vi "ProdaNG.Example.GetTestSteps.vi"() -> ()   [LabVIEW 2016]
uses:
  Controls/ProdaNG.Identification.ctl
  Controls/ProdaNG.TestStep.ctl
  Controls/ProdaNG.ProcessStep.ctl
  Controls/ProdaNG.Process.ctl
  Controls/ProdaNG.ProcessStepParam.ctl
  <vilib>/Utility/miscctls.llb/LVRowAndColumnUnsignedTypeDef.ctl
panel:
  in  "ResultStatus":i32(listbox)
  out "Identification":T1
  in  "ButtonUpdate":bool
  in  "ButtonRead":bool
  in  "Results":i32(listbox)
  out "ProcStepParams":T2[](array[typedef])
  out "Process":T3
  out "ProcStep":T4[](array[typedef])
  out "TestSteps":T5[](array[typedef])
  in  "Product Serial Number":string="1160131100027"
  out "ID":T6
  in  "Systems":u16(ring) items=["ADEK1", "ASTV2_P01", "ASTV2_P02", "ASTV2_P03", "ASTV2_P04", "Connection station", "DPI", "EAPU2_AD", "EAPU2_CONN", "EAPU2_MCPV_1", "EAPU2_MCPV_2", "EBAM2", "EBAM3", "EBAM4", "ED01", "ED04", "ED05", "EPS3_RANGE_DMC", "FAVP_1A", "FAVP_1B", "FESTO", "H17", "H20", "H21", "HAPU P01", "HAPU P02", "HAPU P03", "HAPU_P01", "HAPU_P02", "HAPU_P03", "HAPU_P04", "HAPU_P05", "HAPU_P06", "HP1", "HP10", "HP10L", "HP10R", "HP12", "HP13", "HP15", "HP16", "HP17", "HP18", "HP19", "HP2", "HP20", "HP21", "HP22", "HP23", "HP24", "HP25", "HP26", "HP26L", "HP26R", "HP2L", "HP2R", "HP3", "HP34", "HP35", "HP37", "HP38", "HP39", "HP4", "HP50", "HP51", "HP52", "HP6", "HP7", "HP8", "HP88", "HP8L", "HP8R", "HP9", "KEPSE1", "KEPSE2", "KEPSE3", "KEPSE4", "KEPSE5", "LCS02", "LSM101", "LSM102", "LSM103", "LV_MIX_process", "MAD 1.A", "MAD 1.B", "MAD 2.B", "MAD 2.C", "MAD 4.A", "MAD 4.B", "MAD EOL", "MIX_400", "MIX_820", "MIX_821", "MIX_BST3_030", "MIX_BST3_034", "MT001", "MT002", "MT003", "MT004", "MT005", "MT006", "MT009", "MT010", "MT011", "MT012", "MT013", "MT014", "MT015", "MT016", "MT017", "MT018", "MT019", "MT020", "MT021", "MT022", "MT023", "MT024", "MT025", "MTB1", "MTB10", "MTB11", "MTB12", "MTB14", "MTB15", "NI_06", "NI_13", "P01", "P02", "P25", "P25L", "P25R", "P32", "P32L", "P34", "PEPS3Gang1", "PEPS3Gang2", "PLATES1", "PLC01", "PLC01L", "PLC01R", "PLC02", "PLC02L", "PLC02R", "PLC03", "PLC04", "PLC04L", "PLC04R", "PLC06L", "PLC06R", "PLC07", "PLC07L", "PLC07R", "PLC08", "PLC08L", "PLC08R", "PLC09", "PLC09L", "PLC09R", "PLC10", "PLC11", "PLC11L", "PLC11R", "PLC12", "PLC12L", "PLC12R", "PLC13", "PLC13L", "PLC13R", "PLC14", "PLC14L", "PLC14R", "PLC15", "PLC15L", "PLC15R", "PLC16", "PLC16L", "PLC16R", "PLC17", "PLC17L", "PLC17R", "PLC18", "PLC19", "PLC19L", "PLC19R", "PLC20", "PLC21", "PLC22", "PLC23", "PLC24", "PLC25", "PLC254", "PLC25L", "PLC25R", "PLC27", "PLC27L", "PLC27R", "PLC28", "PLC28L", "PLC28R", "PLC29", "PLC29L", "PLC29R", "PLC30", "PLC31", "PLC32", "PLC34L", "PLC34R", "PLC36", "PLC38", "PLC39", "PLC39L", "PLC39R", "PLC40", "PLC40L", "PLC40R", "PLC41", "PLC41L", "PLC41R", "PLC42", "PLC42L", "PLC42R", "PLC43", "PLC44", "PLC44L", "PLC44R", "PLC45", "PLC45L", "PLC45R", "PLC46", "PLC46L", "PLC46R", "PSPS_02", "RAVP_1", "RAVP_100", "RAVP_2", "RAVP_3", "RIG1", "RIG10", "RIG110", "RIG111", "RIG13", "RIG14", "RIG150", "RIG151", "RIG160", "RIG161", "RIG17", "RIG18", "RIG19", "RIG2", "RIG20", "RIG21", "RIG22", "RIG23", "RIG24", "RIG26", "RIG27", "RIG271", "RIG272", "RIG28", "RIG29", "RIG291", "RIG292", "RIG3", "RIG30", "RIG31", "RIG32", "RIG321", "RIG322", "RIG33", "RIG331", "RIG332", "RIG34", "RIG4", "RIG5", "RIG6", "RIG7", "RIG80", "RIG90", "RSS_PLUS_BASIC_05", "RSS_PLUS_BASIC_P01", "RSS_PLUS_BASIC_S02", "SD001", "SD002", "SMV1_A", "SMV1_B", "SMV2_A", "SMV2_B", "SMV_017300_1", "SMV_017300_2", "SMV_021300_1", "SMV_021300_2", "SMV_320_1", "SMV_320_2", "T001", "T002", "T003", "T004", "T005", "T006", "T007", "T008", "T009", "T010", "T011", "T012", "T013", "T014", "T015", "T016", "T017", "T018", "T019", "T020", "T021", "T022", "T023", "T023_1", "T024", "T025", "T026", "T027", "T028", "T029", "T030", "T031", "T032", "T033", "T034", "T035", "T036", "T037", "T038", "T039", "T040", "T041", "T042", "T043", "T044", "T045", "T050", "T051", "T052", "T053", "T054", "T055", "T056", "T057", "T058", "T059", "T060", "T061", "T062", "T063", "T064", "T065", "T066", "T067", "T068", "T069", "T070", "T071", "T072", "T073", "T074", "T075", "T076", "T077", "T078", "T079", "T080", "T081", "T082", "T083", "T084", "T085", "T086", "T087", "T088", "T089", "T090", "T091", "T092", "T093", "T094", "T095", "T096", "T209", "TB01", "TB02", "TB_MTB59", "TB_MTB60", "TCSVCS_P01", "TCSVCS_P02", "TCSVCS_P03", "TCSVCS_P04", "TEBS-E_01", "TEBS-E_02", "TEBS-E_03", "TEBS-E_04", "TEBS-E_05", "TEBS-E_06A", "TEBS-E_06B", "TEBS-E_06C", "TEBS-E_07", "TEBS-E_08", "TEBS-E_09", "TEBS-E_F_P01", "TEBS-E_F_P02", "TEBS-E_F_P03", "TEBS-E_L_P01", "TEBS-E_L_P02", "TEBS-E_L_P03", "TEBS-P01", "TEBS-P02", "TEBS-P03", "TEBS_OT_P1", "TEBS_OT_P2", "TO29", "T_REMAN_COMP_1", "VXI15", "YR1_T001", "YR1_T002", "YR1_T003", "YR1_T004", "YR1_T005", "YR1_T006", "YR1_T007", "YR1_T008", "YR1_T009", "YR1_T010", "YR1_T011", "YR1_T012", "YR1_T013", "YR1_T014", "YR1_T015", "YR1_T016", "unknown"]
  in  "Wabco Number":u16(ring)=3155 items=["0", "0000000002", "0000000003", "0000000004", "0000000005", "0000000009", "0000000010", "0000000012", "0000000013", "0000000091", "0000000092", "0000000093", "0000000094", "0000000095", "0000000111", "0000000112", "0000000113", "0000000910", "0000000911", "0000000920", "0000000921", "0000000923", "0000000930", "0000000931", "0000000940", "0000000990", "0000000991", "0000000992", "1001001009", "1100000000", "1111110610", "1111111110", "1111111111", "1111111112", "1111111113", "1111111114", "1111111115", "1111111116", "1111111117", "1111111119", "1111111150", "1111111190", "1111118050", "1111119999", "1201201200", "1231231230", "1231231231", "1231231232", "1234567890", "1324070012", "1324079202", "1347141250", "2111111111", "2211111111", "2220009980", "2220009990", "2220110090", "2221111111", "2222222220", "2222222221", "2222222222", "2222222230", "2222222250", "2222222260", "2222222310", "2222222320", "2222222360", "2222222410", "2222222430", "2222222490", "2222223330", "2222224440", "2222225000", "2222510030", "2222510070", "2222510080", "2222510090", "2347141250", "3111111110", "3240020010", "3240020160", "3240020210", "3240026660", "3330110000", "3330110010", "3333333331", "3333333333", "3401750002", "3401950002", "3402250002", "3720600220", "3720600620", "3730110000", "3730110010", "3730110020", "3730110030", "3730110040", "3730110050", "3730110060", "3730110070", "3730110080", "3730110090", "3750103000", "3750103010", "3750103020", "3750103140", "3750103170", "3750103180", "3750103320", "3750103330", "3750150040", "3750150050", "3750150260", "3750150680", "3750150720", "3750150730", "3750155120", "4005000700", "4005000707", "4005000810", "4005000817", "4005000820", "4005000828", "4005000830", "4005000870", "4005000880", "4005001020", "4005001030", "4005001050", "4005001111", "4005009252", "4005009999", "4006000100", "4111510090", "4111510092", "4111540040", "4111540042", "4123520162", "4123520270", "4123520272", "4123520300", "4123520302", "4127040010", "4127040040", "4127040050", "4127040080", "4127040087", "4127040089", "4127040090", "4127040130", "4127040132", "412704013R", "4127040150", "4127040159", "4127040180", "4127040230", "4127040240", "4127040242", "4127040270", "4127040272", "4129990114", "4129990115", "4129990118", "4129990125", "4129990135", "4129990145", "4129990175", "4129990185", "4129990305", "4129990325", "4129990335", "4129990504", "4129996252", "4129996504", "4129996604", "4129996614", "4129996804", "4129996814", "4129996824", "4129996834", "4129996844", "4129996854", "4129996904", "4129996914", "4129996924", "4129997302", "4129997312", "4129997322", "4129998002", "4129999504", "4129999524", "4154043122", "4213500010", "4213500610", "4213500720", "4213500800", "4213500810", "4213500820", "4213500830", "4213500840", "4213500850", "4213500860", "4213500870", "4213500880", "4213509272", "4213509282", "4213509302", "4213509312", "4213509322", "4213509342", "4213509352", "4213509930", "4213509999", "4213510000", "4213510010", "4213510510", "4213510700", "4213510750", "4213510960", "4213510970", "4213510980", "4213511300", "4213511310", "4213511320", "4213511330", "4213511350", "4213511360", "4213511370", "4213511380", "4213511400", "4213511440", "4213511510", "4213511520", "4213511530", "4213511540", "4213511550", "4213511560", "4213511650", "4213511660", "4213511670", "4213511710", "4213511719", "4213511720", "4213511730", "4213511740", "4213511750", "4213511760", "4213511770", "4213511780", "4213511790", "4213511840", "4213511860", "4213511870", "4213519382", "4213519392", "4213519402", "4213519980", "4213519990", "4213520820", "4213529202", "4213529800", "4213529880", "4213529900", "4213529910", "4213529920", "4213529930", "4213529940", "4213529950", "4213529960", "4213529970", "4213529980", "4213529990", "4213554524", "4213554532", "4214113000", "4214113010", "4214113020", "4214113040", "4214113050", "4214113060", "4214113080", "4214113090", "4214113110", "4214113140", "4214113150", "4214113160", "4214150022", "4214270002", "4214290020", "4214290030", "4214290050", "4214290060", "4214410002", "4214410030", "4214410130", "4214410200", "4214410500", "4214410600", "4214420000", "4214420002", "4214420080", "4214420130", "4214420170", "4214420180", "4214420530", "4228020134", "4228023010", "4228023018", "4228023090", "4228023098", "4228023100", "4228023108", "4228023200", "4228023208", "4228023250", "4228023258", "4228023260", "4228024020", "4228024210", "4228024218", "4228033270", "4228033280", "4228033288", "4228081060", "4228081068", "4228090002", "4228100002", "4228100012", "4228100022", "4228100032", "4228110002", "4228120000", "4228120002", "4228120008", "4228120020", "4228120028", "4228120104", "4228120114", "4229010164", "4229020104", "4229030134", "4229030164", "4230000000", "4230035020", "4230035080", "4230039110", "4230070190", "4230080050", "4230080070", "4230089160", "4230089170", "4230089190", "4230540000", "4230540010", "4230550000", "4230550010", "4230550060", "4230550080", "4230550500", "4230550530", "4230551000", "4230560000", "4230560010", "4230560040", "4230560060", "4230560080", "4230560500", "4230560530", "4230570002", "4230570010", "4230570030", "4230570070", "4230570080", "4230570100", "4230580010", "4230580020", "4230600000", "4230600040", "4231020120", "4231020150", "4231029000", "4231030050", "4231030100", "4231031000", "4231031180", "4231032960", "4231032980", "4231039000", "4231040020", "4231040060", "4231040070", "4231040100", "4231040200", "4231040500", "4231040530", "4231040930", "4231040990", "4231042910", "4231042980", "4231046060", "4231046070", "4231046080", "4231046100", "4231046120", "4231046130", "4231046180", "4231046300", "4231046310", "4231046320", "4231046340", "4231046350", "4231046360", "4231046530", "4231047000", "4231047010", "4231047100", "4231047110", "4231047120", "4231047130", "4231047150", "4231047160", "4231050040", "4231050200", "4231050210", "4231050220", "4231050310", "4231050320", "4231050420", "4231050430", "4231050720", "4231050740", "4231050840", "4231050850", "4231050890", "4231050910", "4231050940", "4231051030", "4231051110", "4231051180", "4231051210", "4231051230", "4231051250", "4231051260", "4231051300", "4231051310", "4231051340", "4231051350", "4231051990", "4231052920", "4231052960", "4231052970", "4231052980", "4231054060", "4231054070", "4231054080", "4231054090", "4231054100", "4231054140", "4231054160", "4231054170", "4231054500", "4231054510", "4231057000", "4231057010", "4231057020", "4231057030", "4231057040", "4231057050", "4231060020", "4231060030", "4231060040", "4231060050", "4231060410", "4231060460", "4231060470", "4231060570", "4231060580", "4231060700", "4231060710", "4231060810", "4231060880", "4231060900", "4231060950", "4231061030", "4231061040", "4231061060", "4231061150", "4231061180", "4231061250", "4231061260", "4231061300", "4231061350", "4231061360", "4231061440", "4231061500", "4231061510", "4231061520", "4231061600", "4231061700", "4231062010", "4231062020", "4231062070", "4231062080", "4231062100", "4231062920", "4231062930", "4231062940", "4231062950", "4231062970", "4231062980", "4231064020", "4231064030", "4231064060", "4231064070", "4231064080", "4231064090", "4231064100", "4231064170", "4231064210", "4231064220", "4231064230", "4231064260", "4231064280", "4231064300", "4231064500", "4231067000", "4231067010", "4231069050", "4231069250", "4231069260", "4231069320", "4231069600", "4231070070", "4231070080", "4231070100", "4231070310", "4231070320", "4231070500", "4231070600", "4231070900", "4231070980", "4231071110", "4231071120", "4231072980", "4231074020", "4231074030", "4231074040", "4231074060", "4231074070", "4231074080", "4231074100", "4231074110", "4231074160", "4231074170", "4231079220", "4231079300", "4231090010", "4231090020", "4231090030", "4231090070", "4231090080", "4231090100", "4231090130", "4231090200", "4231090220", "4231090230", "4231090700", "4231091010", "4231091020", "4231091180", "4231091200", "4231097000", "4231097010", "4231099000", "4231100010", "4231107100", "4231107110", "4231127100", "4231140000", "4231140010", "4231140020", "4231140030", "4231140080", "4231140100", "4231140110", "4231140300", "4231140400", "4231146000", "4231146100", "4231147100", "4232051000", "4232051010", "4232051050", "4232051060", "4232067000", "4232067010", "4235030000", "4235030010", "4235030100", "4235030110", "4235031800", "4235031810", "4235040010", "4235040020", "4235040030", "4235040120", "4235040130", "4235040140", "4235040200", "4235040210", "4235040240", "4235040300", "4235040810", "4235040900", "4235040910", "4235041000", "4235041010", "4235041100", "4235041300", "4235041800", "4235041810", "4235050000", "4235050010", "4235050020", "4235050040", "4235050070", "4235050080", "4235050140", "4235050150", "4235050200", "4235050210", "4235050220", "4235050230", "4235050240", "4235050500", "4235050510", "4235050600", "4235050610", "4235051800", "4235051810", "4235051900", "4235051910", "4235060010", "4235060020", "4235060030", "4235060060", "4235060070", "4235060080", "4235060090", "4235060140", "4235060150", "4235060200", "4235060210", "4235060220", "4235060230", "4235060240", "4235060250", "4235060260", "4235060270", "4235060310", "4235060400", "4235060420", "4235060430", "4235060500", "4235060501", "4235060510", "4235060520", "4235060530", "4235060540", "4235060550", "4235060560", "4235060570", "4235060600", "4235060610", "4235060620", "4235060630", "4235060640", "4235060650", "4235060720", "4235060810", "4235061000", "4235061010", "4235061020", "4235061030", "4235061040", "4235061041", "4235061200", "4235061210", "4235061220", "4235061230", "4235061240", "4235061300", "4235061310", "4235061400", "4235061401", "4235061410", "4235061420", "4235061430", "4235061431", "4235061500", "4235061510", "4235061600", "4235061610", "4235070000", "4235090050", "4235090060", "4235090070", "4235090080", "4235090100", "4235090110", "4235090120", "4235090130", "4235090200", "4235090210", "4235090220", "4235090230", "4235090240", "4235090250", "4235090260", "4235100010", "4235100100", "4235100200", "4235100210", "4235100240", "4235100250", "4235100260", "4235110100", "4235110110", "4235120010", "4235120100", "4235121800", "4235121810", "4235140000", "4235140030", "4235140040", "4235140060", "4235140100", "4235140200", "4321111111", "4324060012", "4324060022", "4324060032", "4324062222", "4324069202", "4324100000", "4324100002", "4324100012", "4324100022", "4324100030", "4324100040", "4324100042", "4324100050", "4324100052", "4324100070", "4324100080", "4324100200", "4324100210", "4324100220", "4324100230", "4324100260", "4324100270", "4324100310", "4324100330", "4324100340", "4324100350", "4324100360", "4324100380", "4324100410", "4324100420", "4324100500", "4324100640", "4324100660", "4324100670", "4324100690", "4324100720", "4324100730", "4324100740", "4324100750", "4324100760", "4324100790", "4324100800", "4324100830", "4324100870", "4324100900", "4324100910", "4324100920", "4324100950", "4324101020", "4324101040", "4324101060", "4324101100", "4324101110", "4324101120", "4324101130", "4324101140", "4324101150", "4324101160", "4324101170", "4324101180", "4324101200", "4324101210", "4324101220", "4324101230", "4324101270", "4324101310", "4324101340", "4324101350", "4324101440", "4324101620", "4324101660", "4324101670", "4324101910", "4324101920", "4324102000", "4324102010", "4324102020", "4324102040", "4324102160", "4324102210", "4324102500", "4324102620", "4324105522", "4324107200", "4324107350", "4324109070", "4324109312", "4324109322", "4324109332", "4324109352", "4324111600", "4324111670", "4324111680", "4324111690", "4324120010", "4324120020", "4324120030", "4324120040", "4324130010", "4324130020", "4324130030", "4324130060", "4324130070", "4324130090", "4324130300", "4324130320", "4324130330", "4324130660", "4324131020", "4324139202", "4324139232", "4324139242", "4324139252", "4324139292", "4324139302", "4324139312", "4324139322", "4324139332", "4324139342", "4324139999", "4324150000", "4324150002", "4324150030", "4324150050", "4324150060", "4324150080", "4324150090", "4324150100", "4324150120", "4324150130", "4324150150", "4324150160", "4324150170", "4324150190", "4324150220", "4324150240", "4324150280", "4324150290", "4324150300", "4324150320", "4324150330", "4324150370", "4324150380", "4324150390", "4324150500", "4324150590", "4324150620", "4324150690", "4324150720", "4324151240", "4324151380", "4324159210", "4324160010", "4324160020", "4324160030", "4324160040", "4324160110", "4324161110", "4324162220", "4324200000", "4324200020", "4324200030", "4324200080", "4324209202", "4324209212", "4324209222", "4324209242", "4324209252", "4324209262", "4324210000", "4324210002", "4324210020", "4324210030", "4324210070", "4324210080", "4324210090", "4324210100", "4324210110", "4324210120", "4324210140", "4324210190", "4324210200", "4324210210", "4324210220", "4324210240", "4324210250", "4324210260", "4324210280", "4324210290", "4324210300", "4324210320", "4324210340", "4324210350", "4324210370", "4324210380", "4324210390", "4324211280", "4324216666", "4324219202", "4324250070", "4324250080", "4324250090", "4324250100", "4324252000", "4324259202", "4324259212", "4324259222", "4324259232", "4324259242", "4324260010", "4324260110", "4324261110", "4324262220", "4324300022", "4324309202", "4324309232", "4324309242", "4324309252", "4324309262", "4324309272", "4324309492", "4324310002", "4324310022", "4324315512", "4324319232", "4324319242", "4324319252", "4324319302", "4324319312", "4324319322", "4324319332", "4324319342", "4324319352", "4324319362", "4324319372", "4324319382", "4324319402", "4324319422", "4324320002", "4324320012", "4324330020", "4324330030", "4324330050", "4324330060", "4324330070", "4324330080", "4324330090", "4324330100", "4324330110", "4324330120", "4324330130", "4324330140", "4324330180", "4324330200", "4324330220", "4324330230", "4324330240", "4324330620", "4324331080", "4324331110", "4324331120", "4324331130", "4324331910", "4324332000", "4324332010", "4324332016", "4324332020", "4324332050", "4324332060", "4324332090", "4324332170", "4324332180", "4324332190", "4324332200", "4324332230", "4324332250", "4324332730", "4324332740", "4324332780", "4324332790", "4324332800", "4324332810", "4324332960", "4324332970", "4324332980", "4324332990", "4324332997", "4324336667", "4324337770", "4324339202", "4324339212", "4324339222", "4324339232", "4324339242", "4324339990", "4324339997", "4341000000", "4341000200", "4341000209", "4341000210", "4341000220", "4341000230", "4341000240", "4341000250", "4341000260", "4341000270", "4341000280", "4341000290", "4341000320", "4341000330", "4341000339", "4341000340", "4341000349", "4341000350", "4341000370", "4341000380", "4341000390", "4341000430", "4341000470", "4341000479", "4341000480", "4341000489", "4341000490", "4341000499", "4341000510", "4341000519", "4341000800", "4341000820", "4341000830", "4341001170", "4341001210", "4341001219", "4341001220", "4341001229", "4341001230", "4341001239", "4341001240", "4341001249", "4341001250", "4341001259", "4341001260", "4341001269", "4341001270", "4341001279", "4341001280", "4341001289", "4341001300", "4341001301", "4341001305", "4341001309", "4341001310", "4341001319", "4341001330", "4341001360", "4341001390", "4341001430", "4341001440", "4341001449", "4341001500", "4341001510", "4341001520", "4341001530", "4341002110", "4341002200", "4341002210", "4341002220", "4341002230", "4341002240", "4341002250", "4341002260", "4341002270", "4341002279", "4341002280", "4341002289", "4341002290", "4341002300", "4341002309", "4341002310", "4341002320", "4341002329", "4341002330", "4341002340", "4341002349", "4341002350", "4341002360", "4341002430", "4341002440", "4341002450", "4341002460", "4341002490", "4341002499", "4341002510", "4341002530", "4341002539", "4341002540", "4341002560", "4341002570", "4341002590", "4341002600", "4341002610", "4341002620", "4341005040", "4341005050", "4341005070", "4341005080", "4341006000", "4341006010", "4341006020", "4341006030", "4341006039", "4341006040", "4341008880", "4341009900", "4341009910", "4341009970", "4341009990", "4341080000", "4342050012", "4342050210", "4342050260", "4342050270", "4342050280", "4342050300", "4342050310", "4342050320", "4342050330", "4342050500", "4342050510", "4342050600", "4342050610", "4342059980", "4342059990", "4429987202", "4444444444", "4445010000", "4445010010", "4445010040", "4460806062", "4460806072", "4461080850", "4461082010", "4461082040", "4461082060", "4461082080", "4461451154", "4461451222", "4461451223", "4461640220", "4461640340", "4462600202", "4469990002", "4469990012", "4469990042", "4469990052", "4528020000", "4600000001", "4600000002", "4600000003", "4610000000", "4610000010", "4610000030", "4610000110", "4610000120", "4610000160", "4610001110", "4611060002", "4611061000", "4611061020", "4611061027", "4611061060", "4611064780", "4611110000", "4611110002", "4611110010", "4611110020", "4611130010", "4613070022", "4613070042", "4613072000", "4613072007", "4613072020", "4613073990", "4613074190", "4613074390", "4613074580", "4613074670", "4613074750", "4613074757", "4613074790", "4613074797", "4613075200", "4613075210", "4613103620", "4613105500", "4613150000", "4613150010", "4613150020", "4613150022", "4613150030", "4613150032", "4613150033", "4613150040", "4613150041", "4613150042", "4613150052", "4613150060", "4613150070", "4613150080", "4613150120", "4613150140", "4613150170", "4613150180", "4613150190", "4613150210", "4613150220", "4613150260", "4613150270", "4613150340", "4613150360", "4613150410", "4613150420", "4613150430", "4613150440", "4613150470", "4613150480", "4613150490", "4613150500", "4613150520", "4613150530", "4613150550", "4613150580", "4613150590", "4613150600", "4613150610", "4613150630", "4613150640", "4613150650", "4613150680", "4613150690", "4613150700", "4613150710", "4613150730", "4613150740", "4613150760", "4613150770", "4613150780", "4613150820", "4613150830", "4613150860", "4613150890", "4613151070", "4613151500", "4613151510", "4613151530", "4613151540", "4613151550", "4613151610", "4613151800", "4613152390", "4613152450", "4613152500", "4613152530", "4613152540", "4613152580", "4613152610", "4613152630", "4613152640", "4613154430", "4613154500", "4613154550", "4613154590", "4613154600", "4613154610", "4613154630", "4613154640", "4613154670", "4613154700", "4613154760", "4613154790", "4613154820", "4613154860", "4613154890", "4613154900", "4613154910", "4613154950", "4613154951", "4613154970", "4613155000", "4613159022", "4613159042", "4613159052", "4613159062", "4613159072", "4613159082", "4613159092", "4613159142", "4613159152", "4613159162", "4613159172", "4613159182", "4613159202", "4613159212", "4613159222", "4613159232", "4613159242", "4613159252", "4613159262", "4613159272", "4613159302", "4613159312", "4613159322", "4613159332", "4613160020", "4613180000", "4613180010", "4613180020", "4613180030", "4613180050", "4613180060", "4613180090", "4613180140", "4613180150", "4613180160", "4613180190", "4613180220", "4613180230", "4613180240", "4613180250", "4613180260", "4613180280", "4613180290", "4613180300", "4613180340", "4613180350", "4613180360", "4613180380", "4613180400", "4613180470", "4613180490", "4613180500", "4613180510", "4613180530", "4613180560", "4613180570", "4613180580", "4613180590", "4613180700", "4613180710", "4613181010", "4613184850", "4613184860", "4613184940", "4613184950", "4613185010", "4613185020", "4613185030", "4613185500", "4613185510", "4613185520", "4613186010", "4613186030", "4613186038", "4613186040", "4613186048", "4613186050", "4613186060", "4613186090", "4613186098", "4613186110", "4613189202", "4613189212", "4613189222", "4613189242", "4613189252", "4613190012", "4613190022", "4613190032", "4613190042", "4613190052", "4613190062", "4613190072", "4613190080", "4613190082", "4613190092", "4613190110", "4613190180", "4613190280", "4613190320", "4613190880", "4613192500", "4613192600", "4613192620", "4613192630", "4613192640", "4613192700", "4613192710", "4613192720", "4613192730", "4613192740", "4613192750", "4613192800", "4613199002", "4613199012", "4613199022", "4613199032", "4613199052", "4613199072", "4613199082", "4613199092", "4613199102", "4613199112", "4613199122", "4613240002", "4613240010", "4613240060", "4613240080", "4613240090", "4613240120", "4613240180", "4613240187", "4613240220", "4613240270", "4613240310", "4613240340", "4613240390", "4613240400", "4613240410", "4613240420", "4613240430", "4613240460", "4613245200", "4613245220", "4613246202", "4613280000", "4613300030", "4613330000", "4614780000", "4614780070", "4614820110", "4614820120", "4614820130", "4614820950", "4614911007", "4614911020", "4614911027", "4614911580", "4614911587", "4614912740", "4614912747", "4614940130", "4614947000", "4614947010", "4614947020", "4614947030", "4614947040", "4614947050", "4614947060", "4614947070", "4614947080", "4614990002", "4614990050", "4615130000", "4615130007", "4615130008", "4615130009", "4615130010", "4615130019", "4615130020", "4615130027", "4615130028", "4615130030", "4615130090", "4615130100", "4615130200", "4615130210", "4615130211", "4615130212", "4615130219", "4615131111", "4615139000", "4615139010", "4615139212", "4615139222", "4615139998", "4615139999", "4621930012", "4630220200", "4630220210", "4630281120", "4630281130", "4630320012", "4630320200", "4630320220", "4630320230", "4630320260", "4630320290", "4630321200", "4630321260", "4630321300", "4630321360", "4630380002", "4630380030", "4630380090", "4630380110", "4630380120", "4630380130", "4630380150", "4630390002", "4630390050", "4630390060", "4630489202", "4630489212", "4630840000", "4630840002", "4630840007", "4630840012", "4630840020", "4630840022", "4630840030", "4630840100", "4630840105", "4630840107", "4630840109", "4630840200", "4630840207", "4630840208", "4630840209", "4630840290", "4630840310", "4630840311", "4630840317", "4630840318", "4630840319", "4630840410", "4630840419", "4630840420", "4630840429", "4630840500", "4630840509", "4630841000", "4630841005", "4630841009", "4630849202", "4630849999", "4630860000", "4630860010", "4630860200", "4630860210", "4630860220", "4630860230", "4630860240", "4630860400", "4630860410", "4630860430", "4630860600", "4630860610", "4630900100", "4630900120", "4630900200", "4630900201", "4630900208", "4630900209", "4630900210", "4630900220", "4630900230", "4630900232", "4630900237", "4630900238", "4630900239", "4630900250", "4630901230", "4630905000", "4630905010", "4630905020", "4630905030", "4630905040", "4630905050", "4630905090", "4630905091", "4630905092", "4630905098", "4630905100", "4630999999", "4640060000", "4640060002", "4640060007", "4640060010", "4640060012", "4640060020", "4640060027", "4640060030", "4640060040", "4640060050", "4640060060", "4640060070", "4640060110", "4640060120", "4640060127", "4640060128", "4640060130", "4640061000", "4640061007", "4640061010", "4640061018", "4640061020", "4640062010", "4640065000", "4640065200", "4640065400", "4640065800", "4640069202", "4683970012", "4683970030", "4683970038", "4700120000", "4700120007", "4700125202", "4700130002", "4700135002", "4700150002", "4700150012", "4700150020", "4700150022", "4700150032", "4700150042", "4700150052", "4700150060", "4700150062", "4700150072", "4700150082", "4700150090", "4700150100", "4700150110", "4700150170", "4700150510", "4700150520", "4700150540", "4700150550", "4700150900", "4700150920", "4700150960", "4700150970", "4700150980", "4700150990", "4700152010", "4700152030", "4700152140", "4700152150", "4700152170", "4700152180", "4700152210", "4700152230", "4700152520", "4700152530", "4700152540", "4700152550", "4700152560", "4700152570", "4700152580", "4700152590", "4700152610", "4700152630", "4700152650", "4700152670", "4700152690", "4700152710", "4700152730", "4700152750", "4700152770", "4700153000", "4700153009", "4700153010", "4700153019", "4700155000", "4700159002", "4700159012", "4700159022", "4700159032", "4710035300", "4712000000", "4712000052", "4712000072", "4712000080", "4712001020", "4712001100", "4712001130", "4712001140", "4712001170", "4712001230", "4712080000", "4712080002", "4712080060", "4714010092", "4720020092", "4720841000", "4721950090", "4721950110", "4721950150", "4721950160", "4721950180", "4721950250", "4721950310", "4721950311", "4721950330", "4721950340", "4721950350", "4721950370", "4721950380", "4721950390", "4721950410", "4721950430", "4721950440", "4721950460", "4721950480", "4721950488", "4721950510", "4721950518", "4721950540", "4721950550", "4721950560", "4721950580", "4721950588", "4721950660", "4721950710", "4721950720", "4721950730", "4721950970", "4721951080", "4721951100", "4721951108", "4721951140", "4721959202", "4721959212", "4721959222", "4721960200", "4721960220", "4721960250", "4722500000", "4722500030", "4722500050", "4722500070", "4722500080", "4722510010", "4722510230", "4722510240", "4722510270", "4722600050", "4722600060", "4722600110", "4722609900", "4722609990", "4724000550", "4724000700", "4724050010", "4724050020", "4724050030", "4724050040", "4724059202", "4726000010", "4726000220", "4726009990", "4728800000", "4728800002", "4728800004", "4728800009", "4728800010", "4728800014", "4728800019", "4728800020", "4728800024", "4728800029", "4728800040", "4728800044", "4728800048", "4728800049", "4728800200", "4728800209", "4728800210", "4728800219", "4728800230", "4728800238", "4728800239", "4728800240", "4728800249", "4728800300", "4728800304", "4728800307", "4728800309", "4728800310", "4728800314", "4728800319", "4728800320", "4728800324", "4728800328", "4728800329", "4728800500", "4728800509", "4728800520", "4728800529", "4728800550", "4728800559", "4728800600", "4728800609", "4728800610", "4728800619", "4728800620", "4728800629", "4728800640", "4728800649", "4728800650", "4728800659", "4728800700", "4728800709", "4728800710", "4728800719", "4728800720", "4728800729", "4728800730", "4728800740", "4728801000", "4728801009", "4728801030", "4728801039", "4728801040", "4728801049", "4728801050", "4728801060", "4728809202", "4728809212", "4728809222", "4728809232", "4728809242", "4728809252", "4728809262", "4728809272", "4728809322", "4728809332", "4728809990", "4728900010", "4728900020", "4728900030", "4728900200", "4728900209", "4728900210", "4728900219", "4728900220", "4728900229", "4728900300", "4728900307", "4728900310", "4728900320", "4728900329", "4728900400", "4728900409", "4728900410", "4728900419", "4728900500", "4728900509", "4728900600", "4728900610", "4728900700", "4728900760", "4728900800", "4728900803", "4728900809", "4728901110", "4728901120", "4728901127", "4728901130", "4728901137", "4729000010", "4729000020", "4729000080", "4729000090", "4729000120", "4729000130", "4729000140", "4729000210", "4729000220", "4729000300", "4729000320", "4729000330", "4729000340", "4729000500", "4729000510", "4729000530", "4729000539", "4729000540", "4729000550", "4729000560", "4729000570", "4729000580", "4729000590", "4729000600", "4729000610", "4729000620", "4729000630", "4729000640", "4729000650", "4729000670", "4729000730", "4729000740", "4729001010", "4729001020", "4729001040", "4729001050", "4729001100", "4729001120", "4729001130", "4729001140", "4729009222", "4729050600", "4729050609", "4729050700", "4729050705", "4729050709", "4729051070", "4729051079", "4729051080", "4729051085", "4729051089", "4729051090", "4729051099", "4729051100", "4729051109", "4729051110", "4729051115", "4729051119", "4729051120", "4729051129", "4729051140", "4729051145", "4729051149", "4729051160", "4729051169", "4729051180", "4729051189", "4730130000", "4730150800", "4730170000", "4730170002", "4730170010", "4730170050", "4730170300", "4730170310", "4730179980", "4730179990", "4733030000", "4733030001", "4733030003", "4733030009", "4733030010", "4733030019", "4733030020", "4733030021", "4733030029", "4733030030", "4733030039", "4733030040", "4733030050", "4733030060", "4733030070", "4733030270", "4733031003", "4733031111", "4735010000", "4735010010", "4735010040", "4735010050", "4735012010", "4735012020", "4735012030", "4742000010", "4750090000", "4750090040", "4750090050", "4750090070", "4750090080", "4750090090", "4750090100", "4750090120", "4750090130", "4750090140", "4750090150", "4750090210", "4750090220", "4750090260", "4750090270", "4750090310", "4750090320", "4750091500", "4750091510", "4750091520", "4750100000", "4750100002", "4750100010", "4750100012", "4750100020", "4750100022", "4750100030", "4750100040", "4750100050", "4750100060", "4750100070", "4750100080", "4750100090", "4750100100", "4750100110", "4750100120", "4750100130", "4750100140", "4750100150", "4750100160", "4750100170", "4750100210", "4750100240", "4750100250", "4750100260", "4750100270", "4750100320", "4750101010", "4750101020", "4750101030", "4750101110", "4750102000", "4750102001", "4750102005", "4750102009", "4750102010", "4750102011", "4750103000", "4750103001", "4750103009", "4750103010", "4750103011", "4750103020", "4750103021", "4750103030", "4750103031", "4750103040", "4750103041", "4750103050", "4750103051", "4750103060", "4750103061", "4750103070", "4750103071", "4750103080", "4750103081", "4750103090", "4750103091", "4750103100", "4750103101", "4750103110", "4750103111", "4750103120", "4750103121", "4750103130", "4750103131", "4750103140", "4750103141", "4750103160", "4750103161", "4750103170", "4750103171", "4750103180", "4750103181", "4750103185", "4750103220", "4750103221", "4750103240", "4750103241", "4750103250", "4750103251", "4750103270", "4750103271", "4750103280", "4750103281", "4750103290", "4750103291", "4750103300", "4750103301", "4750103310", "4750103311", "4750103320", "4750103321", "4750103330", "4750103331", "4750103339", "4750103340", "4750103341", "4750103350", "4750103351", "4750103360", "4750103370", "4750103380", "4750103390", "4750103400", "4750103410", "4750103420", "4750103430", "4750103440", "4750103450", "4750103460", "4750104000", "4750104001", "4750108880", "4750150002", "4750150010", "4750150012", "4750150030", "4750150040", "4750150041", "4750150050", "4750150051", "4750150070", "4750150090", "4750150100", "4750150140", "4750150150", "4750150154", "4750150160", "4750150180", "4750150200", "4750150260", "4750150261", "4750150269", "4750150280", "4750150281", "4750150300", "4750150310", "4750150320", "4750150327", "4750150330", "4750150331", "4750150350", "4750150360", "4750150364", "4750150370", "4750150371", "4750150374", "4750150380", "4750150390", "4750150391", "4750150400", "4750150410", "4750150440", "4750150450", "4750150460", "4750150470", "4750150480", "4750150490", "4750150540", "4750150550", "4750150560", "4750150570", "4750150580", "4750150590", "4750150600", "4750150609", "4750150610", "4750150611", "4750150614", "4750150615", "4750150616", "4750150620", "4750150630", "4750150631", "4750150640", "4750150650", "4750150660", "4750150670", "4750150680", "4750150700", "4750150710", "4750150720", "4750150721", "4750150730", "4750150731", "4750150740", "4750150750", "4750150760", "4750150770", "4750150780", "4750150800", "4750150810", "4750150811", "4750150820", "4750150821", "4750150830", "4750150831", "4750150840", "4750150841", "4750150850", "4750150851", "4750150860", "4750150861", "4750150870", "4750150871", "4750150880", "4750150881", "4750151010", "4750151020", "4750153000", "4750153001", "4750154000", "4750154001", "4750155000", "4750155001", "4750155010", "4750155030", "4750155100", "4750155120", "4750155127", "4750155128", "4750156610", "4750159000", "4750159792", "4750159802", "4750159970", "4750159980", "4750159990", "4750159999", "4750190000", "4750200020", "4750200050", "4750200060", "4750200110", "4756040022", "4756040100", "4756040110", "4756040120", "4756040130", "4756040410", "4756040430", "4756040500", "4756041100", "4756041120", "4756041210", "4757000042", "4757001220", "4757001260", "4757002200", "4757004020", "4757004037", "4757009212", "4757010002", "4757010010", "4757010050", "4757010070", "4757010092", "4757010120", "4757010130", "4757010200", "4757010210", "4757017122", "4757020000", "4757020002", "4757020012", "4757020200", "4757020220", "4757100000", "4757100012", "4757100022", "4757100030", "4757100042", "4757100060", "4757100070", "4757100080", "4757100110", "4757100120", "4757100130", "4757100140", "4757100160", "4757100200", "4757100210", "4757100220", "4757100240", "4757100250", "4757100270", "4757100280", "4757100290", "4757100310", "4757100320", "4757100330", "4757100350", "4757100360", "4757100390", "4757100400", "4757100410", "4757100420", "4757100440", "4757100450", "4757100460", "4757100570", "4757100750", "4757100820", "4757101210", "4757101220", "4757101240", "4757101280", "4757101290", "4757101300", "4757101310", "4757101340", "4757101350", "4757101360", "4757101440", "4757101560", "4757107112", "4757110002", "4757110012", "4757110020", "4757110030", "4757110040", "4757110060", "4757110070", "4757110090", "4757110100", "4757110110", "4757110120", "4757110130", "4757110170", "4757110200", "4757110210", "4757110220", "4757110230", "4757110240", "4757110250", "4757110260", "4757110270", "4757110280", "4757110290", "4757110300", "4757110320", "4757110330", "4757110340", "4757110360", "4757110370", "4757110380", "4757110390", "4757110400", "4757110410", "4757110420", "4757110450", "4757110460", "4757110470", "4757110510", "4757110520", "4757110580", "4757110600", "4757110680", "4757110720", "4757110740", "4757110750", "4757110760", "4757110870", "4757110890", "4757110900", "4757110940", "4757110960", "4757110970", "4757110980", "4757110990", "4757111080", "4757111100", "4757111110", "4757111130", "4757111140", "4757111150", "4757111170", "4757111180", "4757111190", "4757111200", "4757111210", "4757111220", "4757111250", "4757111260", "4757111270", "4757111280", "4757111340", "4757111420", "4757111430", "4757111450", "4757111460", "4757111480", "4757111490", "4757111500", "4757111540", "4757111550", "4757111590", "4757120000", "4757120002", "4757120040", "4757127102", "4757130000", "4757130002", "4757130020", "4757135000", "4757135010", "4757137102", "4757140002", "4757140012", "4757145000", "4757145010", "4757145030", "4757145040", "4757145090", "4757145100", "4757145110", "4757145302", "4757145312", "4757146000", "4757146030", "4757150002", "4757155000", "4757155010", "4757155050", "4757155070", "4757155110", "4757155130", "4757155140", "4757200010", "4757200020", "4757200030", "4757200040", "4757200050", "4757200060", "4757200070", "4757200080", "4757205000", "4757210000", "4757210010", "4757210020", "4757210030", "4757210040", "4757210050", "4757210060", "4757210070", "4757210080", "4757210090", "4757210110", "4757210170", "4757210180", "4757210190", "4757215000", "4757215010", "4757215030", "4757220000", "4757230000", "4757230010", "4757230030", "4758000042", "4758003010", "4758003017", "4758003030", "4758003060", "4758003070", "4770100020", "4770100030", "4770100050", "4770100060", "4770100070", "4770102304", "4770102314", "4770104706", "4770106504", "4770106514", "4770106524", "4770106534", "4770109362", "4800030300", "4800030305", "4800030307", "4800030309", "4800030320", "4800030330", "4800030340", "4800030351", "4800030361", "4800030370", "4800030375", "4800030379", "4800030380", "4800030390", "4800030400", "4800030410", "4800030420", "4800030431", "4800030440", "4800030470", "4800030500", "4800030520", "4800030530", "4800030551", "4800030561", "4800030580", "4800030590", "4800030600", "4800030610", "4800030620", "4800030631", "4800030640", "4800030650", "4800030670", "4800100140", "4800100150", "4801020100", "4801020102", "4801020107", "4801020109", "4801020132", "4801020140", "4801020147", "480102014R", "4801020150", "4801020152", "4801020157", "4801020160", "4801020200", "4801020207", "4801020300", "4801020310", "4801020320", "4801020330", "4801020340", "4801020350", "4801020360", "4801020400", "4801020409", "4801020410", "4801020419", "4801020600", "4801020610", "4801020620", "4801020630", "4801020640", "4801020650", "4801020660", "4801020700", "4801020709", "4801020710", "4801020719", "4801020800", "4801020840", "4801029342", "4801030080", "4801030110", "4801030120", "4801030130", "4801030140", "4801030150", "4801030160", "4801030220", "4801030240", "4801030250", "4801030330", "4801030350", "4801030410", "4801030420", "4801030430", "4801030610", "4801030630", "4801030660", "4801039212", "4801070000", "4801100010", "4802020010", "4802020040", "4802020050", "4802020070", "4802020080", "4802020090", "4802020100", "4802020120", "4802020180", "4802021000", "4802021120", "4802022000", "4802029090", "4802029212", "4802040020", "4802040300", "4802040305", "4802040309", "4802040310", "4802040320", "4802047242", "4802049202", "4802049999", "4802050010", "4802050100", "4802051010", "4802051020", "4802051030", "4802051040", "4802051060", "4802051080", "4802059212", "4802070010", "4802072020", "4802079202", "4809050109", "4809050119", "4809990124", "4809990164", "4809990504", "5555555550", "5555555551", "5555555554", "5555555555", "5750200110", "5750200120", "6666666666", "7777777700", "7777777710", "7777777750", "7777777770", "7777777777", "8440118120", "8810118120", "8840000000", "8840057740", "8840078190", "8840114000", "8840114001", "8840114002", "8840115220", "8840115550", "8840115570", "8840116940", "8840118090", "8840118120", "8840125750", "8840126140", "8840126141", "8840126142", "8840126143", "8840134700", "8840135720", "8840135730", "8840135760", "8840135770", "8840135780", "8840135830", "8840137811", "8840138711", "8840140680", "8840140690", "8840140700", "8840146000", "8840146210", "8840146880", "8840146980", "8840149490", "8840149580", "8840149590", "8840149630", "8840149999", "8840151650", "8840151660", "8840153151", "8840153190", "8840154000", "8840156600", "8840162050", "8840163200", "8840167400", "8840173000", "8840173240", "8840186550", "8840187820", "8840187821", "8840213000", "8840320200", "8840320260", "8840323330", "8840323340", "8840584410", "8840587390", "8840588980", "8840588981", "8840588982", "8840588983", "8840589000", "8840601000", "8840601010", "8840621400", "8845100070", "8888888880", "8888888888", "8942600402", "8942600742", "8949997782", "8990538044", "9000009110", "9119996252", "9119996254", "9119996272", "9119996274", "9119997332", "9119997504", "9121120000", "9121120009", "9121120010", "9121140000", "9121140009", "9121420000", "9121420009", "9121420010", "9121510000", "9122100000", "9122100122", "9122108002", "9125101030", "9125101032", "9125101040", "9125101042", "9125120040", "9125120049", "9125120060", "9125120062", "9125120080", "9125120089", "9125120190", "9125120220", "9125120280", "9125120290", "9125120292", "9125120300", "9125140010", "9125140019", "9125140030", "9125140040", "9125140060", "9125140070", "9125140080", "9125140100", "9125220000", "9125220010", "9125270000", "9125420010", "9125420019", "9125420020", "9125420060", "9125420080", "9125510020", "9125510050", "9125510070", "9129986934", "9129990135", "9129994304", "9129994314", "9129996222", "9129996224", "9129996272", "9129996274", "9129997302", "9228000150", "9250000000", "9254207500", "9254207507", "9254207510", "9254207520", "9254207530", "9254207540", "9254210370", "9254211410", "9254211420", "9254215400", "9254217500", "9254217507", "9254217510", "9254217520", "9254221200", "9254221220", "9254221230", "9254221500", "9254221510", "9254263300", "9254291760", "9254291770", "9254300300", "9254300307", "9254300350", "9254300357", "9254300360", "9254300367", "9254300410", "9254300660", "9254300667", "9254310320", "9254310330", "9254310337", "9254310340", "9254310350", "9254310357", "9254310360", "9254310370", "9254310377", "9254310380", "9254310387", "9254310400", "9254310407", "9254310410", "9254310417", "9254310420", "9254310470", "9254310480", "9254310630", "9254310637", "9254311000", "9254311007", "9254314210", "9254314220", "9254314227", "9254314230", "9254314600", "9254314900", "9254314907", "9254319100", "9254319110", "9254320200", "9254320210", "9254320220", "9254320227", "9254321120", "9254321130", "9254321140", "9254321150", "9254321157", "9254321160", "9254321167", "9254321170", "9254321177", "9254321180", "9254321187", "9254321200", "9254321210", "9254321300", "9254324400", "9254324407", "9254324410", "9254324420", "9254340000", "9254600270", "9254600320", "9254601000", "9254601010", "9254612900", "9254612910", "9254613200", "9254613210", "9254613300", "9254613310", "9254613500", "9254613510", "9254614700", "9254614710", "9254615000", "9254615010", "9254615020", "9254615030", "9254640120", "9254640130", "9254640140", "9254640150", "9254640160", "9254640400", "9254644500", "9254644507", "9254644510", "9254644517", "9254644520", "9254644527", "9254645000", "9254645010", "9254660100", "9254680320", "9254700000", "9254700010", "9254800100", "9254800110", "9254800610", "9254802920", "9254810000", "9254810010", "9254810140", "9254810150", "9254810160", "9254810170", "9254810240", "9254810250", "9254810260", "9254810270", "9254810280", "9254810300", "9254810310", "9254810320", "9254810330", "9254810340", "9254810400", "9254810410", "9254810500", "9254810510", "9254810600", "9254810700", "9254811000", "9254811010", "9254811020", "9254811030", "9254811040", "9254811080", "9254811100", "9254811110", "9254811120", "9254811130", "9254811140", "9254811150", "9254811160", "9254811170", "9254811180", "9254811200", "9254811210", "9254811220", "9254811230", "9254811240", "9254811250", "9254811500", "9254811560", "9254811570", "9254811600", "9254811610", "9254811630", "9254811640", "9254811810", "9254811910", "9254812300", "9254812310", "9254812320", "9254812700", "9254812710", "9254812720", "9254813100", "9254813110", "9254813120", "9254813130", "9254813140", "9254813200", "9254813260", "9254813270", "9254813280", "9254813300", "9254813310", "9254813320", "9254813330", "9254813340", "9254813350", "9254813360", "9254813370", "9254813380", "9254813420", "9254813430", "9254813440", "9254813450", "9254813460", "9254813470", "9254813480", "9254813600", "9254813610", "9254813620", "9254813630", "9254813760", "9254814200", "9254814210", "9254814240", "9254814250", "9254814300", "9254814310", "9254814500", "9254814900", "9254814910", "9254814920", "9254814930", "9254840100", "9254840110", "9254840200", "9254840210", "9254840220", "9254840230", "9254840260", "9254840340", "9254840400", "9254840410", "9254849600", "9254860100", "9254860110", "9254860120", "9254860500", "9254860600", "9254860800", "9254860810", "9254861040", "9254861050", "9254861060", "9254861100", "9254861110", "9254863050", "9254864000", "9254864010", "9254880000", "9254880010", "9254880130", "9254880140", "9254880150", "9254880200", "9254880210", "9254880220", "9254880230", "9254880300", "9254880400", "9254880410", "9254880600", "9254880610", "9254900200", "9254900210", "9254900220", "9254900230", "9254900400", "9254900410", "9254900420", "9254900700", "9254901030", "9254901040", "9254909010", "9254909020", "9254909050", "9254909060", "9254910050", "9254910600", "9254910610", "9254910620", "9254910630", "9254910780", "9254911030", "9254911040", "9254911050", "9254911060", "9254911070", "9254911080", "9254911170", "9254911180", "9254911300", "9254911330", "9254911600", "9254911620", "9254912400", "9254912700", "9254914300", "9254914310", "9254919000", "9254919010", "9254920010", "9254920012", "9254920200", "9254922000", "9254922090", "9254922100", "9254922140", "9254922150", "9254922210", "9254922310", "9254922320", "9254927220", "9254927230", "9254929020", "9254929030", "9254949100", "9254949110", "9254960010", "9254960040", "9254990002", "9254990030", "9254990040", "9254990110", "9254990120", "9254990300", "9254990310", "9254990340", "9254990700", "9254990710", "9254990800", "9254990810", "9254990820", "9254990830", "9255349600", "9255349610", "9255349620", "9255349640", "9255349890", "9255809810", "9324000002", "9324000010", "9324000020", "9324000030", "9324000050", "9324000060", "9324000080", "9324000100", "9324000130", "9324000140", "9324000160", "9324000170", "9324000180", "9324000210", "9324000230", "9324000240", "9324000310", "9324000330", "9324000550", "9324006660", "9324007000", "9324008010", "9324008020", "9324008050", "9324008060", "9324009001", "9324009002", "9324009010", "9324009020", "9324009050", "9324009060", "9324009101", "9324009130", "9324009140", "9324009202", "9324019010", "9324019020", "9324019050", "9324019060", "9324019140", "9324019160", "9325000040", "9325000050", "9325000060", "9325000061", "9325000070", "9325000071", "9325000130", "9325000140", "9325000141", "9325000150", "9325000160", "9325000210", "9325000380", "9325000390", "9325000400", "9325000550", "9325000680", "9325000681", "9325000880", "9325000930", "9325000940", "9325001010", "9325001070", "9325001100", "9325001110", "9325050010", "9325050020", "9325100010", "9325100020", "9325100021", "9325100030", "9325100031", "9325100040", "9325100049", "9325100050", "9325100060", "9325100062", "9325100090", "9325100100", "9325100110", "9325100500", "9325109202", "9325109242", "9325109252", "9325109352", "9325109392", "9325109412", "9325109422", "9325109442", "9325109452", "9325109462", "9325109492", "9325109512", "9325109522", "9325109552", "9325109612", "9325109622", "9325109672", "9329055032", "9341111110", "9347010002", "9347020000", "9347020012", "9347020020", "9347020050", "9347020052", "9347020082", "9347020092", "9347020400", "9347020410", "9347020420", "9347020450", "9347020470", "9347020820", "9347021000", "9347021010", "9347021011", "9347021100", "9347021200", "9347021210", "9347021220", "9347021910", "9347021920", "9347022100", "9347022200", "9347022210", "9347022230", "9347022400", "9347022500", "9347022510", "9347022520", "9347022600", "9347022610", "9347022700", "9347022710", "9347023000", "9347023020", "9347023200", "9347023220", "9347023230", "9347023300", "9347023400", "9347023420", "9347023800", "9347023810", "9347023870", "9347023880", "9347026660", "9347029002", "9347029012", "9347029032", "9347050020", "9347050030", "9347050040", "9347050050", "9347050051", "9347050060", "9347050080", "9347050090", "9347050100", "9347050110", "9347050130", "9347050140", "9347050150", "9347050210", "9347050220", "9347050230", "9347050310", "9347050320", "9347051110", "9347059212", "9347140010", "9347140030", "9347140040", "9347140060", "9347140100", "9347140120", "9347140140", "9347140160", "9347140190", "9347140270", "9347140300", "9347141090", "9347141100", "9347141110", "9347141190", "9347141230", "9347141250", "9347141260", "9347141280", "9347141320", "9347141340", "9347141370", "9347141380", "9347141400", "9347141450", "9347141460", "9347143020", "9347143200", "9347144000", "9347144010", "9347145550", "9347146660", "9347147400", "9347149212", "9347149222", "9347149232", "9347149242", "9349010052", "9611060000", "9611060002", "9630000010", "9630000020", "9630000030", "9630010012", "9630060002", "9650010010", "9650010170", "9650010180", "9650010410", "9650010420", "9650010450", "9650010460", "9650010470", "9650010480", "9650010500", "9650010510", "9650010520", "9650010530", "9650010540", "9650010550", "9650019282", "9650019999", "9701501000", "9701509999", "9710020000", "9710020010", "9710020012", "9710020020", "9710020032", "9710020033", "9710020040", "9710020042", "9710020050", "9710020052", "9710020062", "9710020082", "9710020099", "9710021500", "9710021501", "9710021502", "9710021507", "9710021510", "9710021520", "9710021527", "9710021530", "9710021570", "9710022000", "9710022030", "9710023000", "9710023007", "9710023010", "9710023030", "9710023037", "9710023040", "9710023050", "9710023070", "9710023077", "9710023080", "9710025310", "9710025317", "9710025330", "9710025337", "9710025470", "9710025700", "9710025800", "9710026200", "9710027000", "9710027007", "9710027010", "9710027017", "9710027020", "9710027030", "9710027040", "9710028050", "9710029000", "9710029001", "9710029002", "9710029003", "9710029007", "9710029008", "9710029009", "9710029017", "9710029020", "9710029027", "9710029100", "9710029107", "9710029109", "9710029110", "9710029117", "9710029120", "9710029127", "9710029130", "9710029137", "9710029200", "9710029210", "9710029220", "9710029232", "9710029242", "9710029252", "9710029990", "9719719710", "9730010002", "9730010003", "9730010022", "9730010032", "9730010052", "9730010062", "9730010100", "9730010130", "9730010180", "9730010200", "9730010210", "9730010218", "9730010300", "9730010310", "9730010320", "9730012100", "9730012110", "9730012200", "9730012210", "9730020000", "9730020032", "9730020042", "9730020043", "9730020052", "9730020053", "9730020062", "9730020070", "9730020082", "9730020092", "9730020100", "9730020130", "9730020200", "9730020220", "9730020510", "9730020700", "9730024020", "9730024030", "9730024040", "9730024050", "9730024060", "9730024090", "9730024180", "9730024190", "9730024220", "9730024230", "9730024250", "9730024300", "9730024500", "9730025000", "9730025010", "9730025030", "9730025050", "9730025200", "9730025210", "9730025220", "9730025230", "9730025240", "9730025250", "9730025270", "9730025280", "9730025300", "9730025320", "9730025350", "9730025380", "9730025390", "9730025440", "9730025700", "9730026200", "9730030000", "9730030002", "9730030020", "9730030060", "9730030070", "9730030080", "9730030100", "9730030120", "9730030130", "9730060000", "9730060010", "9730060020", "9730060030", "9730060031", "9730060033", "9730060034", "9730060035", "9730060037", "9730069920", "9730090002", "9730090010", "9730090012", "9730090020", "9730090040", "9730090050", "9730090060", "9730090070", "9730090090", "9730090100", "9730090130", "9730090140", "9730090150", "9730090160", "9730090180", "9730090220", "9730090230", "9730090250", "9730090260", "9730091000", "9730091200", "9730093000", "9730100002", "9730110000", "9730110002", "9730110010", "9730110012", "9730110020", "9730110022", "9730110040", "9730110050", "9730110052", "9730110060", "9730110062", "9730110072", "9730110080", "9730110090", "9730110100", "9730110110", "9730110380", "9730110500", "9730110630", "9730110670", "9730111000", "9730111010", "9730111030", "9730111050", "9730111060", "9730111070", "9730111090", "9730111100", "9730111110", "9730112000", "9730112010", "9730112030", "9730112050", "9730112060", "9730112080", "9730112500", "9730112510", "9730112520", "9730113000", "9730113010", "9730119990", "9735000000", "9735000002", "9735000012", "9735000030", "9735000042", "9735000060", "9735000140", "9735000180", "9735000280", "9735000300", "9735000310", "9735000340", "9735000380", "9735000390", "9735000420", "9735000440", "9735000450", "9735000470", "9735000510", "9735000530", "9735000550", "9735000570", "9735000590", "9750020010", "9750020012", "9750020030", "9750020040", "9750020050", "9750020170", "9750020710", "9750020720", "9750020730", "9750090010", "9750090020", "9750090030", "9750090040", "9750090050", "9750091010", "9750091110", "9750092010", "9750092110", "9750099990", "9760001000", "9760001010", "9760001020", "9760001030", "9760001050", "9760001060", "9760001070", "9760001080", "9760001090", "9760001100", "9760001110", "9760001120", "9762001000", "9762001010", "9970110010", "9970110040", "9970112500", "9970112510", "9970113000", "9971111110", "9975000000", "9990110000", "9990110010", "9990110020", "9990110040", "9990110080", "9990110090", "9990110100", "9990110110", "9990110380", "9990110500", "9990110630", "9990110670", "9990112000", "9990112010", "9990112030", "9990112050", "9990112060", "9990112080", "9990112500", "9990112510", "9990112520", "9990113000", "9990113010", "9991001000", "9995000280", "9995000340", "9995000420", "9995000590", "9999909150", "9999990209", "9999990309", "9999991039", "9999999260", "9999999999", "unknown"]
  in  "Connection string":string="lcptb/lcptb@PRODA_WPL"
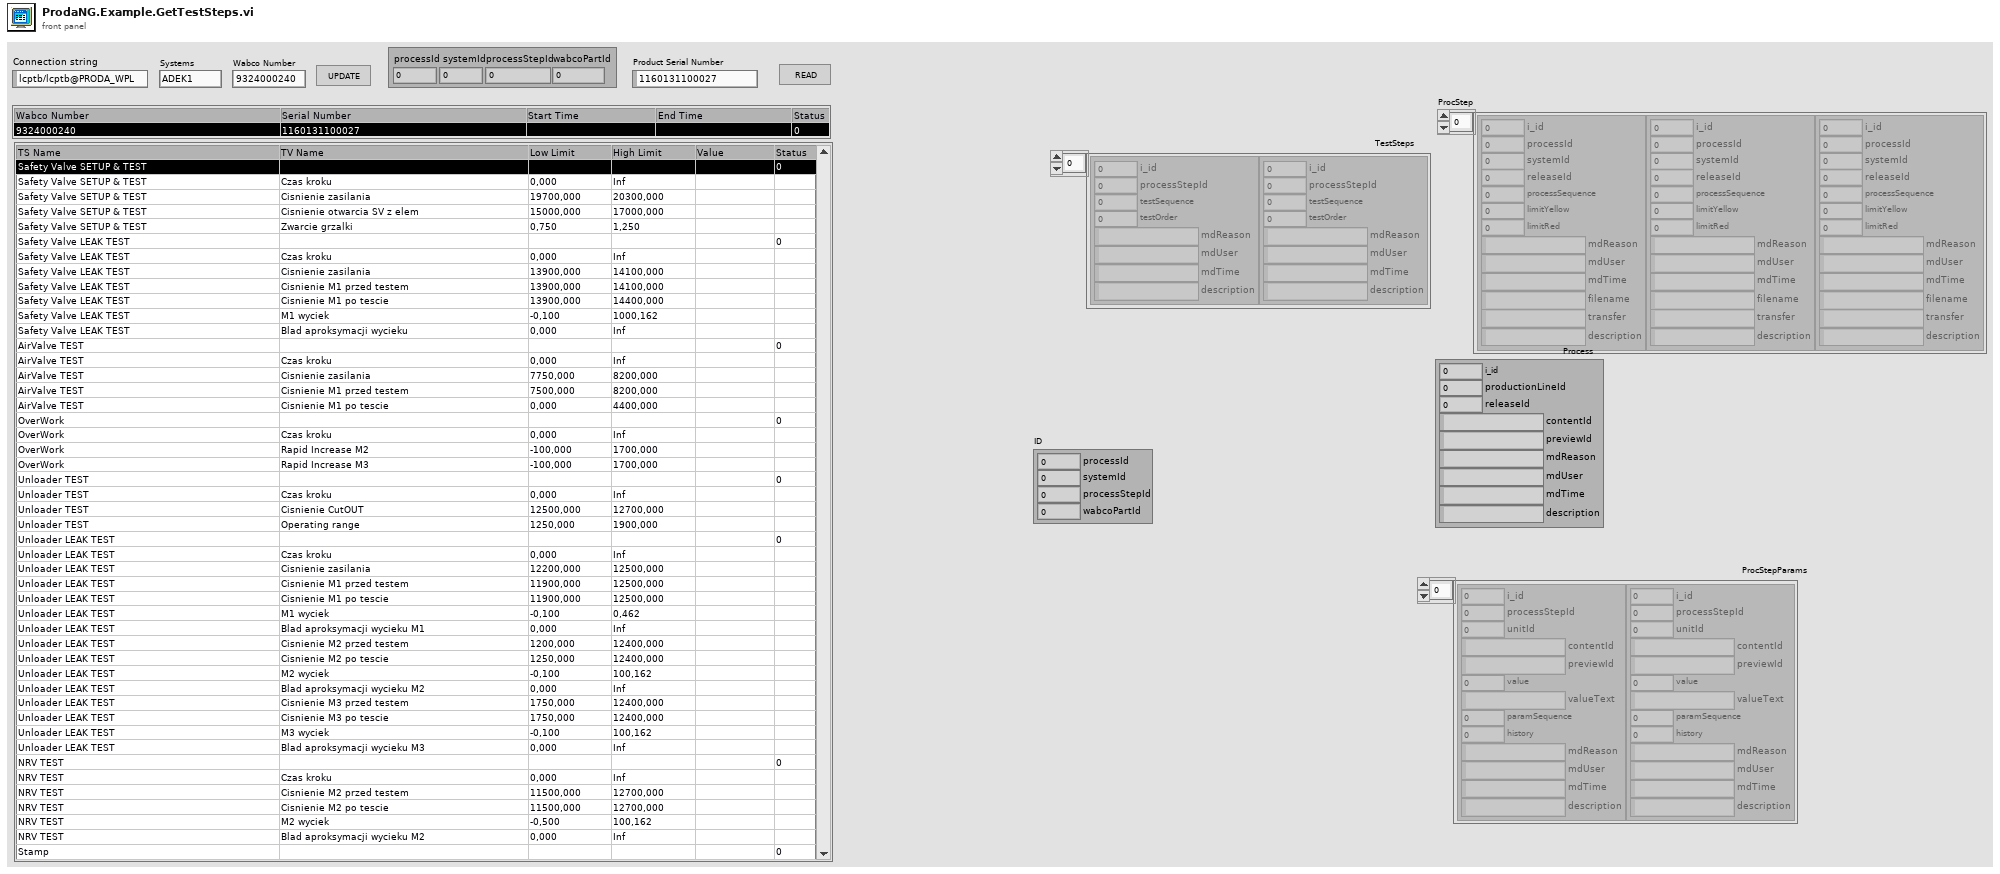
[diagram p1: front panel]
types:
  T1 = cluster{"processId":i32, "systemId":i32, "processStepId":i32, "wabcoPartId":i32}
  T2 = typedef "ProdaNG.ProcessStepParam.ctl" = cluster{"i_id":i32, "processStepId":i32, "unitId":i32, "contentId":string, "previewId":string, "value":dbl, "valueText":string, "paramSequence":i32, "history":i32, "mdReason":string, "mdUser":string, "mdTime":string, "description":string}
  T3 = typedef "ProdaNG.Process.ctl" = cluster{"i_id":i32, "productionLineId":i32, "releaseId":i32, "contentId":string, "previewId":string, "mdReason":string, "mdUser":string, "mdTime":string, "description":string}
  T4 = typedef "ProdaNG.ProcessStep.ctl" = cluster{"i_id":i32, "processId":i32, "systemId":i32, "releaseId":i32, "processSequence":i32, "limitYellow":dbl, "limitRed":dbl, "mdReason":string, "mdUser":string, "mdTime":string, "filename":string, "transfer":string, "description":string}
  T5 = typedef "ProdaNG.TestStep.ctl" = cluster{"i_id":i32, "processStepId":i32, "testSequence":i32, "testOrder":i32, "mdReason":string, "mdUser":string, "mdTime":string, "description":string}
  T6 = typedef "ProdaNG.Identification.ctl" = cluster{"processId":i32, "systemId":i32, "processStepId":i32, "wabcoPartId":i32}
  T7 = enum8{"Enabled", "Disabled", "Disabled and Grayed Out"}
  T8 = typedef "LVRowAndColumnUnsignedTypeDef.ctl" = cluster{"Row":u32, "Column":u32}
  T9 = typedef "ProdaNG.WabcoPart.ctl" = cluster{"i_id":i32, "workCenterId":i32, "contentId":string, "previewId":string, "mdReason":string, "mdUser":string, "mdTime":string, "productName":string, "wabcoNumber":string}
  T10 = typedef "ProdaNG.System.ctl" = cluster{"i_id":i32, "description":string}
  T11 = typedef "ProdaNG.Product.ctl" = cluster{"c_id":string, "wabcoPartId":i32, "serialNumber":string, "comment":string, "individual":i32, "crProcessStepId":i32, "mdProcessStepId":i32, "crTime":string, "mdTime":string}
  T12 = typedef "ProdaNG.ProcessResult.ctl" = cluster{"c_id":string, "productId":string, "processId":i32, "statusId":i32, "startTime":string, "endTime":string}
  T13 = typedef "ProdaNG.ProcessStepResult.ctl" = cluster{"c_id":string, "processResultId":string, "processStepId":i32, "statusId":i32, "operatorId":i32, "startTime":string, "endTime":string}
  T14 = typedef "ProdaNG.TestStepResult.ctl" = cluster{"c_id":string, "processStepResultId":string, "testStepId":i32, "statusId":i32}
  T15 = typedef "ProdaNG.TestValue.ctl" = cluster{"i_id":i32, "testStepId":i32, "releaseId":i32, "unitId":i32, "contentId":string, "previewId":string, "maximum":dbl, "minimum":dbl, "valueText":string, "testValueSequence":i32, "history":i32, "mdReason":string, "mdUser":string, "mdTime":string, "description":string}
  T16 = typedef "ProdaNG.TestValueResult.ctl" = cluster{"c_id":string, "testStepResultId":string, "testValueId":i32, "result":dbl, "statusId":i32, "contentId":string}
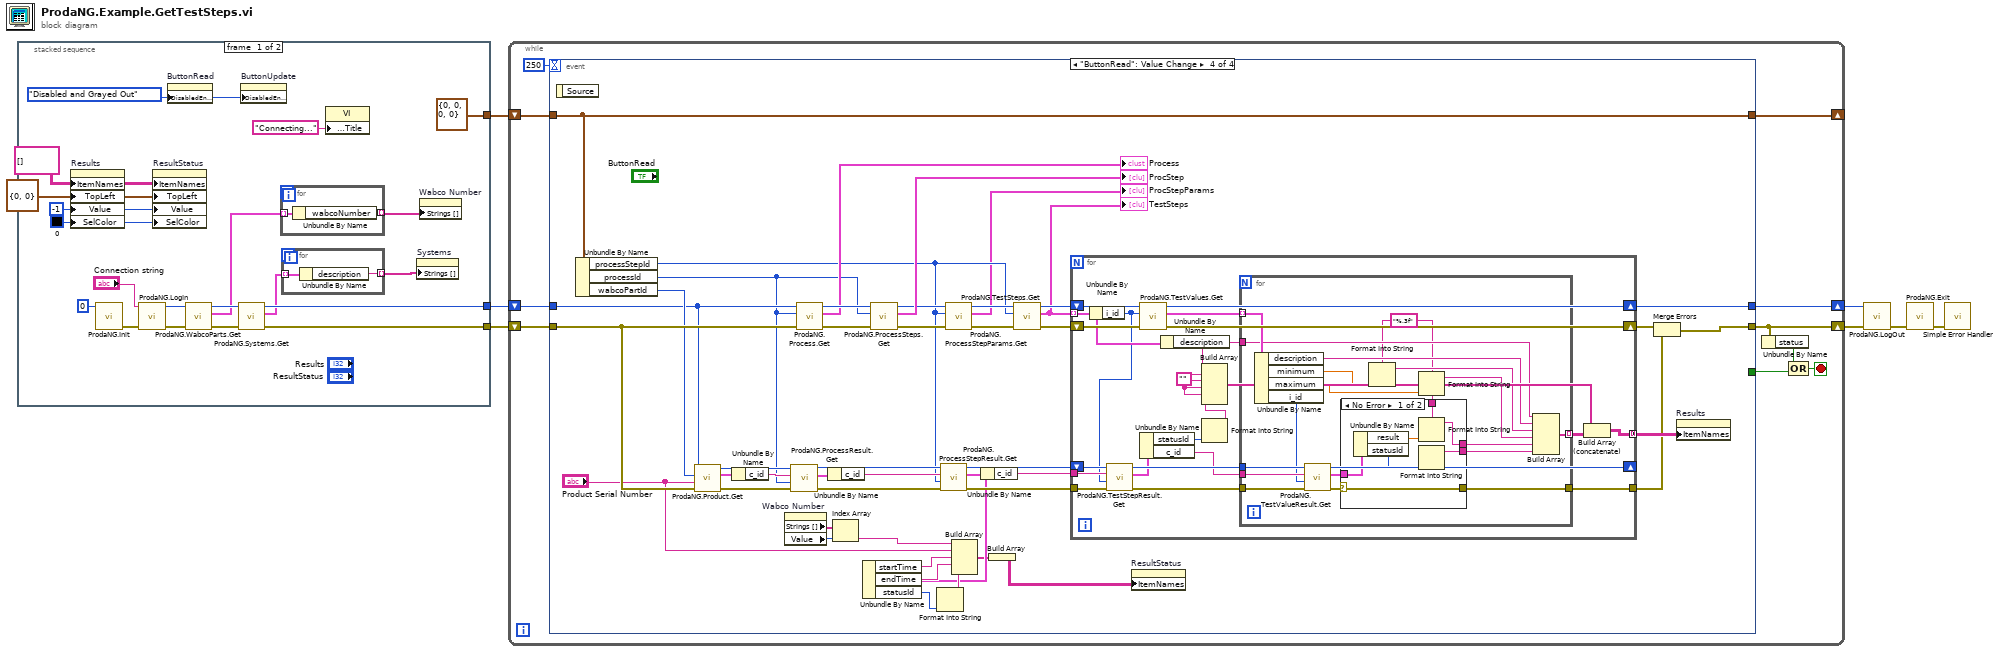
[diagram p0: block diagram]
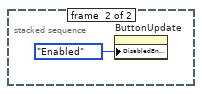
[diagram p2: hidden frame]
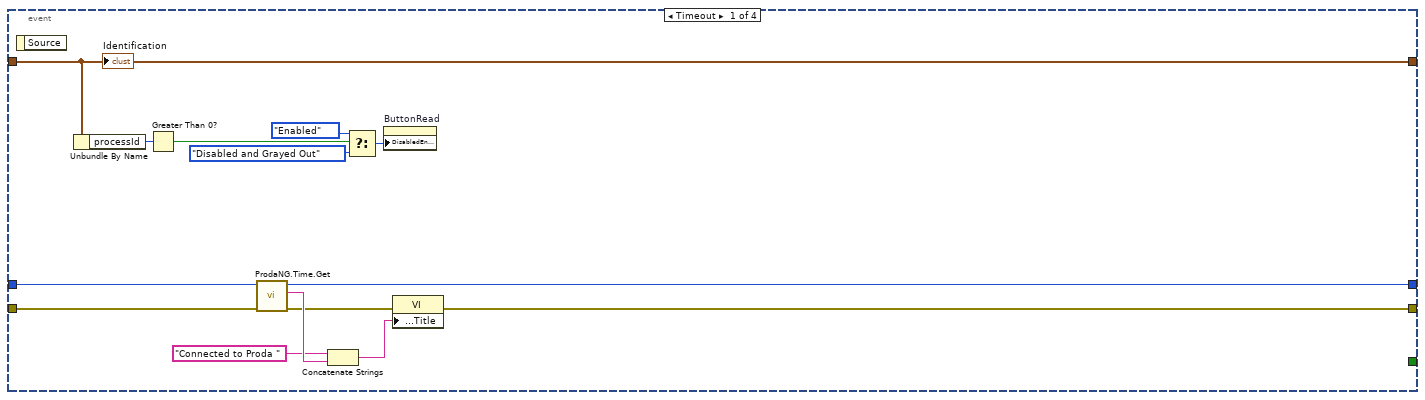
[diagram p3: hidden frame]
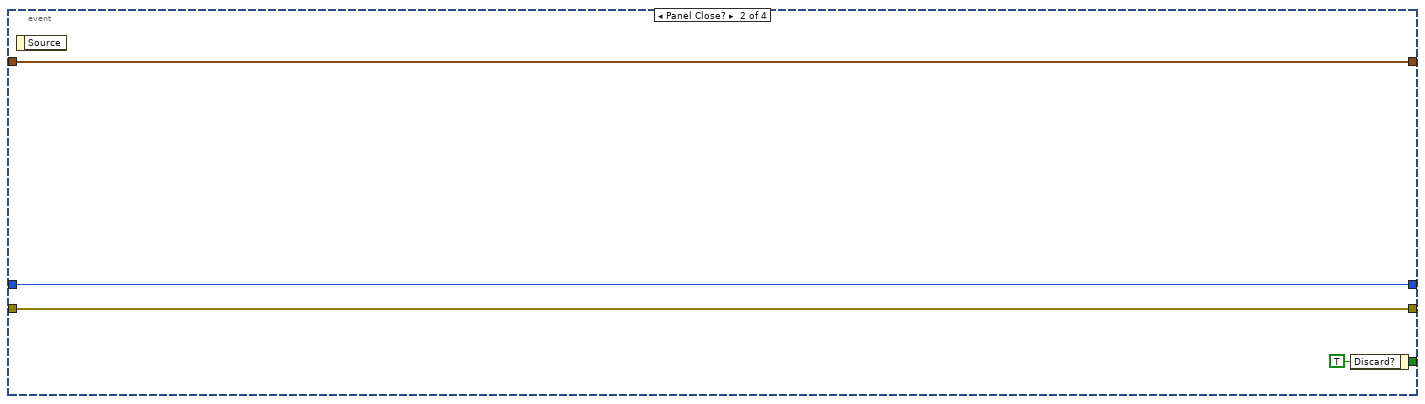
[diagram p4: hidden frame]
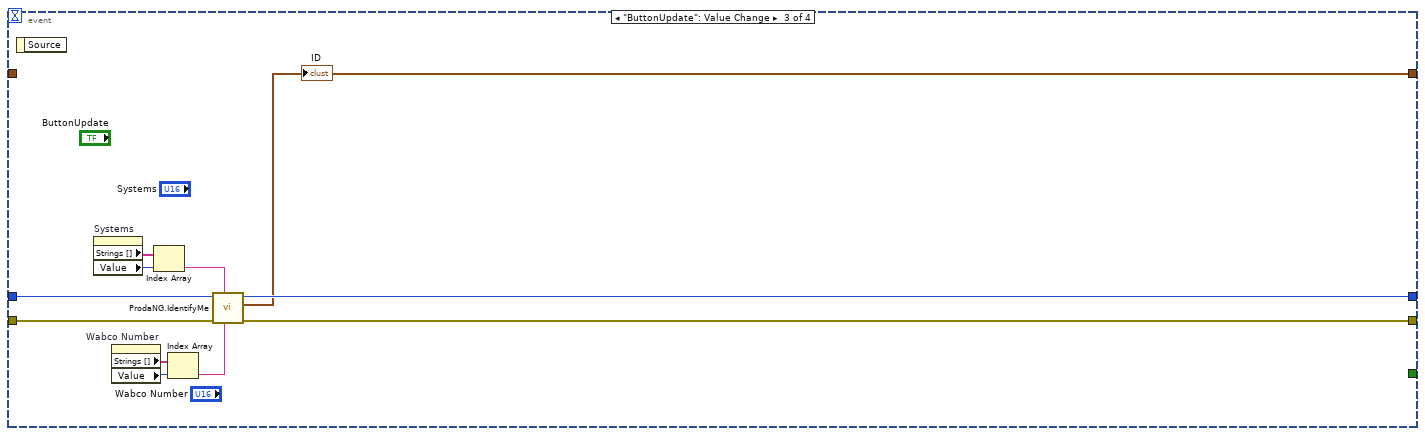
[diagram p5: hidden frame]
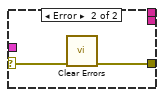
[diagram p6: hidden frame]
diagram:
  n1 = stacked-sequence {
    tunnel: [w22 _] -> w4
    tunnel: [w15 _] -> w3
    tunnel: [T6 {"processId"=0, "systemId"=0, "processStepId"=0, "wabcoPartId"=0} ("Identification") _] -> w2
    frame #0 {
      w13 = T7."Disabled and Grayed Out" ("Disabled")
      w9 = u32 0
      w8 = -1 ("Results")
      w10 = T8 {"Row"=0, "Column"=0} ("Top Left Visible Cell")
      w11 = string[][] [] ("Item Names")
      n2 = property on="Results" class="MCListbox (strict)"("ItemNames"=w11, "TopLeft"=w10, "Value"=w8, "SelColor"=w9) -> ()  [unwired: 2 in, 2 out]
      n3 = call "ProdaNG.Init.vi"("numContexts (0: unlimited)"=0 ("numContexts")) -> ("error out"=w27:errorcluster)  [unwired: 10 in]
      n4 = call "ProdaNG.LogIn.vi"("error in"=w27, "ConnectionString"="Connection string") -> ("error out"=w20:errorcluster, "dbHandle"=w24:i32)  [unwired: 7 in, 1 out]
      n5 = property on="ResultStatus" class="MCListbox (strict)"("ItemNames"=w11, "TopLeft"=w10, "Value"=w8, "SelColor"=w9) -> ()  [unwired: 2 in, 2 out]
      n6 = property on="ButtonRead" class="Bool"("DisabledEnum"=w13) -> ()  [unwired: 2 in, 2 out]
      n7 = call "ProdaNG.WabcoParts.Get.vi"("error in (no error)"=w20, "dbHandleIn"=w24) -> ("error out"=w21:errorcluster, "WabcoParts"=w17:T9[], "dbHandle"=w23:i32)  [unwired: 7 in]
      n8 = call "ProdaNG.Systems.Get.vi"("error in (no error)"=w21, "dbHandleIn"=w23) -> ("error out"=w15:errorcluster, "Systems"=w19:T10[], "dbHandle"=w22:i32)  [unwired: 7 in]
      n9 = property on="ButtonUpdate" class="Bool"("DisabledEnum"=w13) -> ()  [unwired: 2 in, 2 out]
      n10 = for {
        tunnel: w17 -> [w29] mode=indexing
        tunnel: [w28] -> w16 mode=indexing
        n11 = Unbundle By Name(w29) -> ("wabcoNumber"=w28:string)
      }
      n12 = for {
        tunnel: w19 -> [w31] mode=indexing
        tunnel: [w30] -> w18 mode=indexing
        n13 = Unbundle By Name(w31) -> ("description"=w30:string)
      }
      n14 = property class="VI"("Front Panel.Title"="Connecting..." ("Front Panel Window:Title")) -> ()  [unwired: 2 in, 2 out]
      n15 = property on="Systems" class="Ring (strict)"("Strings []"=w18) -> ()  [unwired: 2 in, 2 out]
      n16 = property on="Wabco Number" class="Ring (strict)"("Strings []"=w16) -> ()  [unwired: 2 in, 2 out]
    }
    frame #1 {
      n17 = property on="ButtonUpdate" class="Bool"("DisabledEnum"=T7."Enabled" ("Disabled")) -> ()  [unwired: 2 in, 2 out]
    }
  }
  n18 = while {
    shift-right: [w36] -> w5
    shift-left: w3 -> [w41]
    shift-right: [w42] -> w6
    shift-left: w4 -> [w40]
    shift-right: [w38] -> _
    shift-left: w2 -> [w37]
    stop <- w33 stop-if-true
    n19 = event shown="[3] \"ButtonRead\": Value Change" {
      selector: _ -> [_ _ _ _]
      dyn-events: _ -> [_ _ _ _]
      timeout: 250 -> [_ _ _ _]
      tunnel: [w54 w57 w68 w105] -> w42
      tunnel: w41 -> [w55 w58 w70 w103]
      tunnel: w40 -> [w56 w57 w71 w97]
      tunnel: [w43 w58 w69 w89] -> w36
      tunnel: [w48 w60 w67 w83] -> w38
      tunnel: w37 -> [w48 w60 _ w83]
      tunnel: [_ w59 _ _] -> w35
      event Timeout {
        n20 = event-data() -> ()  [unwired: 1 in, 1 out]
        n21 = Unbundle By Name(w48) -> ("processId"=w53:i32)
        n22 = Greater Than 0?(x=w53) -> (x > 0?=w52:bool)
        n23 = call "ProdaNG.Time.Get.vi"("error in"=w55, "dbHandleIn"=w56) -> ("error out"=w44:errorcluster, "timeStr"=w47:string, "dbHandle"=w54:i32)  [unwired: 5 in, 1 out]
        n24 = Concatenate Strings("Connected to Proda " ("string"), w47) -> (w46:string)
        n25 = Select(t=T7."Enabled" ("Disabled"), s=w52, f=T7."Disabled and Grayed Out" ("Disabled")) -> (s? t:f=w51:T7)
        n26 = property on="ButtonRead" class="Bool"("DisabledEnum"=w51) -> ()  [unwired: 2 in, 2 out]
        n27 = property class="VI"(error in=w44, "Front Panel.Title"=w46) -> (error out=w43:errorcluster)  [unwired: 1 in, 1 out]
        "Identification" <- w48
      }
      event Panel Close? {
        w59 = TRUE ("Discard?")
        n28 = event-data() -> ()  [unwired: 1 in, 1 out]
        n29 = event-data("Discard?"=w59) -> ()  [unwired: 1 in, 1 out]
      }
      event "ButtonUpdate": Value Change {
        n30 = event-data() -> ()  [unwired: 1 in, 1 out]
        n31 = property on="Systems" class="Ring (strict)"() -> ("Strings []"=w63:string[], "Value"=w62:u16)  [unwired: 2 in, 2 out]
        n32 = property on="Wabco Number" class="Ring (strict)"() -> ("Strings []"=w65:string[], "Value"=w66:u16)  [unwired: 2 in, 2 out]
        n33 = Index Array(array=w63, index=w62) -> (element=w61:string)
        n34 = Index Array(array=w65, index=w66) -> (element=w64:string)
        n35 = call "ProdaNG.IdentifyMe.vi"("wabcoNumber"=w64, "systemName"=w61, "error in"=w70, "dbHandleIn"=w71) -> ("error out"=w69:errorcluster, "Identification"=w67:T6, "dbHandle"=w68:i32)  [unwired: 5 in]
        "ID" <- w67
      }
      event "ButtonRead": Value Change {
        n36 = event-data() -> ()  [unwired: 1 in, 1 out]
        n37 = Unbundle By Name(w83) -> ("processStepId"=w92:i32, "processId"=w96:i32, "wabcoPartId"=w102:i32)
        n38 = call "ProdaNG.Product.Get.vi"("error in (no error)"=w103, "serialNumber"="Product Serial Number", "wabcoPartId"=w102, "dbHandle"=w97) -> ("error out"=w101:errorcluster, "Product"=w99:T11, "dbHandle out"=w98:i32)  [unwired: 4 in, 1 out]
        n39 = Unbundle By Name(w99) -> ("c_id"=w100:string)
        n40 = property on="Wabco Number" class="Ring (strict)"() -> ("Strings []"=w76:string[], "Value"=w77:u16)  [unwired: 2 in, 2 out]
        n41 = call "ProdaNG.ProcessResult.Get.vi"("error in (no error)"=w101, "processId"=w96, "productId"=w100, "dbHandle"=w98) -> ("error out"=w93:errorcluster, "ProcessResult"=w87:T12, "dbHandle out"=w94:i32)  [unwired: 4 in, 1 out]
        n42 = call "ProdaNG.Process.Get.vi"("error in (no error)"=w103, "processId"=w96, "dbHandleIn"=w97) -> ("error out"=w115:errorcluster, "Process"=→"Process":T3, "dbHandle"=w114:i32)  [unwired: 5 in, 1 out]
        n43 = Unbundle By Name(w87) -> ("c_id"=w95:string)
        n44 = Index Array(array=w76, index=w77) -> (element=w75:string)
        n45 = call "ProdaNG.ProcessSteps.Get.vi"("error in (no error)"=w115, "processId"=w96, "dbHandleIn"=w114) -> ("error out"=w111:errorcluster, "ProcSteps"=→"ProcStep":T4[], "dbHandle"=w112:i32)  [unwired: 6 in]
        n46 = call "ProdaNG.ProcessStepResult.Get.vi"("error in (no error)"=w93, "processStepId"=w92, "processResultId"=w95, "dbHandle"=w94) -> ("error out"=w91:errorcluster, "ProcessStepResult"=w74:T13, "dbHandle out"=w90:i32)  [unwired: 4 in, 1 out]
        n47 = Unbundle By Name(w74) -> ("startTime"=w81:string, "endTime"=w80:string, "statusId"=w79:i32)
        n48 = Format Into String(w79) -> (resulting string=w78:string)  [unwired: 3 in, 1 out]
        n49 = call "ProdaNG.ProcessStepParams.Get.vi"("error in (no error)"=w111, "processStepId"=w92, "dbHandleIn"=w112) -> ("error out"=w110:errorcluster, "ProcStepParams"=→"ProcStepParams":T2[], "dbHandle"=w109:i32)  [unwired: 6 in]
        n50 = Build Array(w75, "Product Serial Number", w81, w80, w78) -> (w73:string[])
        n51 = Unbundle By Name(w74) -> ("c_id"=w88:string)
        n52 = Build Array(w73) -> (w72:string[][])
        n53 = call "ProdaNG.TestSteps.Get.vi"("error in (no error)"=w110, "processStepId"=w92, "dbHandleIn"=w109) -> ("error out"=w107:errorcluster, "TestSteps"=w106:T5[], "dbHandle"=w108:i32)  [unwired: 6 in]
        "TestSteps" <- w106
        n54 = for {
          tunnel: w106 -> [w129] mode=indexing
          shift-right: [w136] -> w105
          shift-left: w108 -> [w137]
          shift-right: [w135] -> w104
          shift-left: w107 -> [w138]
          shift-right: [w132] -> _
          shift-left: w90 -> [w134]
          tunnel: w88 -> [w133]
          tunnel: [w121] -> w86 mode=concatenating
          tunnel: w91 -> [w126]
          tunnel: [w128] -> w84
          w122 = ""
          n55 = Unbundle By Name(w129) -> ("i_id"=w118:i32)
          n56 = call "ProdaNG.TestStepResult.Get.vi"("error in (no error)"=w126, "testStepId"=w118, "processStepResulttId"=w133, "dbHandle"=w134) -> ("error out"=w127:errorcluster, "TestStepResult"=w117:T14, "dbHandle out"=w132:i32)  [unwired: 4 in, 1 out]
          n57 = call "ProdaNG.TestValues.Get.vi"("error in (no error)"=w138, "testStepId"=w118, "dbHandleIn"=w137) -> ("error out"=w135:errorcluster, "TestStepValues"=w131:T15[], "dbHandle"=w136:i32)  [unwired: 6 in]
          n58 = Unbundle By Name(w117) -> ("statusId"=w124:i32, "c_id"=w119:string)
          n59 = Unbundle By Name(w129) -> ("description"=w125:string)
          n60 = Format Into String(w124) -> (resulting string=w123:string)  [unwired: 3 in, 1 out]
          n61 = Build Array(w125, w122, w122, w122, w122, w123) -> (w120:string[])
          n62 = for {
            tunnel: w119 -> [w156]
            tunnel: w132 -> [w155]
            tunnel: w127 -> [w154]
            tunnel: w131 -> [w153] mode=indexing
            tunnel: [w149] -> w130 mode=indexing
            tunnel: w125 -> [w146]
            tunnel: [w144] -> w128
            w139 = "%.3f" ("format string")
            n63 = Unbundle By Name(w153) -> ("description"=w147:string, "minimum"=w143:dbl, "maximum"=w140:dbl, "i_id"=w152:i32)
            n64 = call "ProdaNG.TestValueResult.Get.vi"("error in (no error)"=w154, "testValueId"=w152, "testStepResultId"=w156, "dbHandle"=w155) -> ("error out"=w145:errorcluster, "TestValueResult"=w151:T16)  [unwired: 5 in, 1 out]
            n65 = case shown="No Error" w145 {
              selector: w145 -> [w158 w165]
              tunnel: w151 -> [w163 _]
              tunnel: [w161 _] -> w150
              tunnel: [w160 _] -> w148
              tunnel: [w158 w164] -> w144
              tunnel: w139 -> [w157 _]
              frame No Error {
                n66 = Unbundle By Name(w163) -> ("result"=w162:dbl, "statusId"=w159:i32)
                n67 = Format Into String(format string=w157, w162) -> (resulting string=w160:string)  [unwired: 2 in, 1 out]
                n68 = Format Into String(w159) -> (resulting string=w161:string)  [unwired: 3 in, 1 out]
              }
              frame Error {
                n69 = call <vilib>:"Clear Errors.vi"("error in (no error)"=w165) -> ("error out"=w164:errorcluster)  [unwired: 5 in, 1 out]
              }
            }
            n70 = Format Into String(format string=w139, w143) -> (resulting string=w141:string)  [unwired: 2 in, 1 out]
            n71 = Format Into String(format string=w139, w140) -> (resulting string=w142:string)  [unwired: 2 in, 1 out]
            n72 = Build Array(w146, w147, w141, w142, w148, w150) -> (w149:string[])
          }
          n73 = Build Array (concatenate)(w120, w130) -> (w121:string[][])
        }
        n74 = property on="ResultStatus" class="MCListbox (strict)"("ItemNames"=w72) -> ()  [unwired: 2 in, 2 out]
        n75 = Merge Errors(w104, w84) -> (w89:errorcluster)
        n76 = property on="Results" class="MCListbox (strict)"("ItemNames"=w86) -> ()  [unwired: 2 in, 2 out]
      }
    }
    n77 = Unbundle By Name(w36) -> ("status"=w34:bool)
    n78 = Compound Arithmetic op=OR(w34, w35) -> (w33:bool)
  }
  n79 = call "ProdaNG.LogOut.vi"("error in"=w5, "dbHandleIn"=w6) -> ("error out"=w7:errorcluster)  [unwired: 9 in]
  n80 = call "ProdaNG.Exit.vi"("error in (no error)"=w7) -> ("error out"=w1:errorcluster)  [unwired: 10 in]
  n81 = call <vilib>:"Simple Error Handler.vi"("error in (no error)"=w1) -> ()  [unwired: 4 in, 5 out]
